vi "Error.vi"(8 "error in":errorcluster, 11 "Data":variant) -> (0 "error out":errorcluster)   [LabVIEW 2018, in "Testing UI 2.lvlib"]
doc: "This subVI enqueues the named action in to the communications queue along with the input data."
uses:
  Testing UI 2.lvlib
  Private Controls/Module Data.ctl
  Private Controls/Module Action.ctl
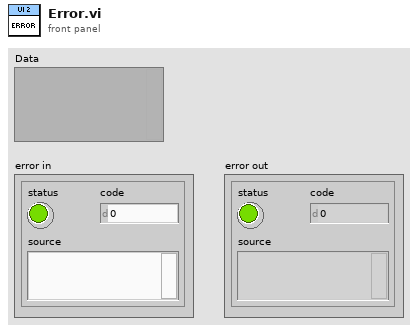
[diagram p1: front panel]
types:
  T1 = typedef "Testing UI 2.lvlib/Module Data.ctl" = cluster{"Data":variant, "Action":T2}
  T2 = typedef "Testing UI 2.lvlib/Module Action.ctl" = enum8{"Init", "Error", "Exit", "HideShow FP", "Send Control Vals", "Update Indicators", "Load APU Setup", "Update APU Name", "Threshold ALERT", "Update Borders", "Update Test Information"}
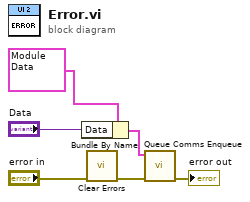
[diagram p0: block diagram]
diagram:
  n1 = Bundle By Name(cluster=T1 {"Data"=variant, "Action"=enum."Error"} ("element"), "Data"="Data") -> (w5:T1)
  n2 = call <vilib>:"Clear Errors.vi"("error in (no error)"="error in") -> ("error out"=w1:errorcluster)  [unwired: 5 in, 1 out]
  n3 = call "Queue Comms Enqueue.vi"("error in (no error)"=w1, "element"=w5) -> ("error out"=→"error out":errorcluster)  [unwired: 9 in]
